vi "Pulse Enable.vi"(8 "error in (no error)":errorcluster, 9 "Value":u8 format="%.0x", 10 "VISA resource name in":refnum<visa-resource-name>, 11 "LCD-I2C in":refnum<class "LCD-I2C.lvclass">) -> (0 "error out":errorcluster, 2 "VISA resource name":refnum<visa-resource-name>, 3 "LCD-I2C out":refnum<class "LCD-I2C.lvclass">)   [LabVIEW 2023, in "CTI-Visa-DeviceLib.lvlib" / "LCD-I2C.lvclass"]
uses:
  LCD-I2C.lvclass
  a2e71dc7-0b7b-4f59-a042-649d55d41a05.vi
  98a5ab1e-28ec-43ee-9f7f-0fcc924d4414.vi
  LCD-I2C.lvclass/LCD-I2C.ctl
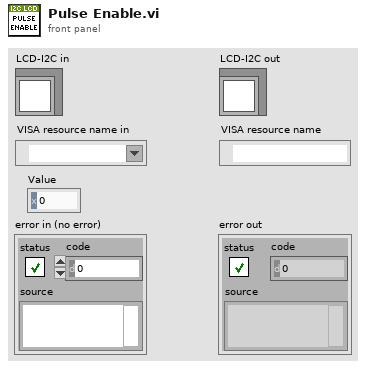
[diagram p1: front panel]
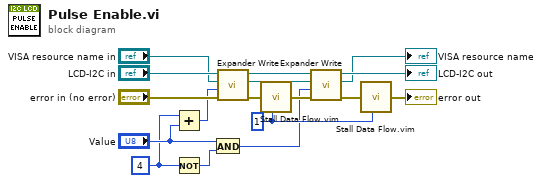
[diagram p0: block diagram]
diagram:
  w4 = u32 1 ("milliseconds to wait")
  w3 = u8 4
  n1 = Add(x=w3, y="Value") -> (x+y=w9:u8)
  n2 = Not(x=w3) -> (.not. x?=w1:u8)
  n3 = And(x="Value", y=w1) -> (x .and. y?=w2:u8)
  n4 = call "Expander Write.vi"("error in (no error)"="error in (no error)", "Value"=w9, "VISA resource name in"="VISA resource name in", "LCD-I2C in"="LCD-I2C in") -> ("error out"=w15:errorcluster, "VISA resource name"=w8:refnum<visa-resource-name>, "LCD-I2C out"=w12:refnum<class "LCD-I2C.lvclass">)  [unwired: 5 in]
  n5 = call "Stall Data Flow.vim"("value in"=w15, "milliseconds to wait"=w4) -> ("value out"=w17:errorcluster)  [unwired: 1 out]
  n6 = call "Expander Write.vi"("error in (no error)"=w17, "Value"=w2, "VISA resource name in"=w8, "LCD-I2C in"=w12) -> ("error out"=w13:errorcluster, "VISA resource name"=→"VISA resource name":refnum<visa-resource-name>, "LCD-I2C out"=→"LCD-I2C out":refnum<class "LCD-I2C.lvclass">)  [unwired: 5 in]
  n7 = call "Stall Data Flow.vim"("value in"=w13, "milliseconds to wait"=w4) -> ("value out"=→"error out":errorcluster)  [unwired: 1 out]
